vi "ExQSnapNframeSeq.vi"() -> ()   [LabVIEW 2010]
uses:
  Open-Close/CamHandle.vi
panel:
  out "Collecting":bool
  out "ADC Gain":u32
  out "ADC Offset":u32
  out "Pixel time":u32
  in  "OK Button":bool
  out "Readout Port":u32
  in  "ADC Gain":u32
  out "ADC Speed (Khz)":u32
  in  "ReadOut Port":u32 max=1 step=1
  in  "Trigger Edge":u32(ring)=1 items=["", "Positive (leading) edge", "Negative (falling) Edge"]
  in  "Trigger/Timing Mode":u32(ring)=1 items=["N/A", "FreeRun/Timed", "Single Trigger (PM only)", "Ext Sync/Strobed", "Bulb (PM only)", "Variable (PM only)", "Flash Mode (PM only)"]
  in  "Y End":u32=128 min=1 step=1
  in  "Y Start":u32=1 min=1 step=1
  in  "X Bin":u32=1 min=1 step=1
  in  "X End":u32=128 min=1 step=1
  in  "Y Bin":u32=1 min=1 step=1
  in  "X Start":u32=1 min=1 step=1
  in  "Number of Images":u32=50 min=1 step=1
  in  "Temperature":dbl format="%.2f"
  in  "Exposure":dbl min=0.0 step=0.001 format="%.3f"
  out "error out":errorcluster
  in  "error in (no error)":errorcluster
  # "ExCoolSnapNframeSeq:\nThis example sets up the camera with a given ROI, and \ncollects into a file \"number of Images\"  set by user. The \nImages are also displayed.\nNote: not all cameras support nframe.\nThis also shows how to setup the Cascade for nframe \nUsing Sequence mode"
  # "NOTICE\n\nTHIS VI USES A GLOBAL CAMERA HANDLE\n\nTHE VI EXOPENGLOBALCAM.VI MUST BE\nRUN AT THE START OF THE WORK SESSION.\nTHE CAMERA WILL REMAIN OPENED.\n\nTHE VI EXCLOSEGLOBALCAM.VI MUST\nBE RUN BEFORE LEAVING LABVIEW."
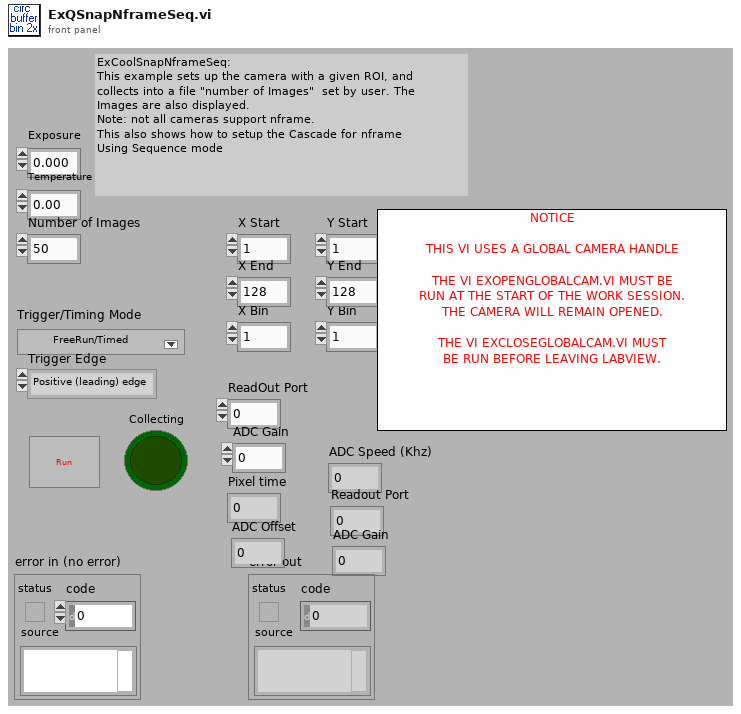
[diagram p1: front panel]
types:
  T1 = cluster{"X Start":u32, "X End":u32, "X Bin":u32, "Y Start":u32, "Y End":u32, "Y Bin":u32}
  T2 = cluster{"acquire focus mode":u32, "Exposure":dbl, "Number of Images":u32, "Software accumulation":u32}
  T3 = cluster{"Camera Handle":u32, "File Handle":u32, "Display Handle":u32, "Image Handle":u32}
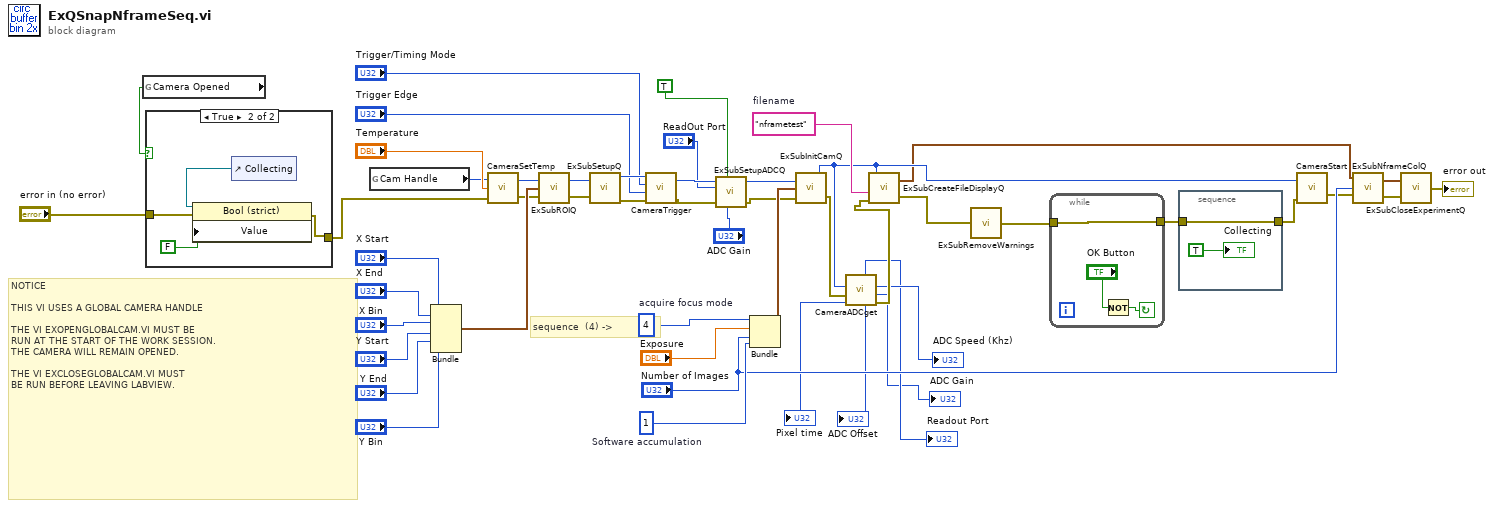
[diagram p0: block diagram]
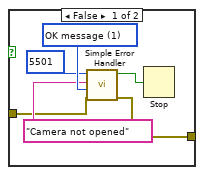
[diagram p2: hidden frame]
diagram:
  w44 = u32 4  # acquire focus mode
  w43 = u32 1  # Software accumulation
  w50 = "nframetest"  # filename
  # "NOTICE\n\nTHIS VI USES A GLOBAL CAMERA HANDLE\n\nTHE VI EXOPENGLOBALCAM.VI MUST BE\nRUN AT THE START OF THE WORK SESSION.\nTHE CAMERA WILL REMAIN OPENED.\n\nTHE VI EXCLOSEGLOBALCAM.VI MUST\nBE RUN BEFORE LEAVING LABVIEW."
  # "sequence  (4) ->"
  n1 = global read "CamHandle.vi" "Camera Opened"() -> (w7:bool)
  n2 = case shown="True" w7 {
    tunnel: [w55 w59] -> w5
    tunnel: "error in (no error)" -> [w51 w60]
    frame False {
      w56 = u16 1 items=["no dialog", "OK message", "continue or stop message"] ("type of dialog (OK msg:1)")
      n3 = call <vilib>:"Simple Error Handler.vi"("error code (no error:0)"=5501, "error source (\" \")"="Camera not opened", "type of dialog (OK msg:1)"=w56, "error in (no error)"=w51) -> ("error?"=w53:bool, "error out"=w55:errorcluster)  [unwired: 1 in, 3 out]
      n4 = Stop(stop? (T)=w53) -> ()
    }
    frame True {
      n5 = control-ref of="Collecting"() -> (w58:refnum<vi>)
      n6 = property class="Bool (strict)"(reference=w58, error in=w60, "Value"=FALSE) -> (error out=w59:errorcluster)  [unwired: 1 out]
    }
  }
  n7 = global read "CamHandle.vi" "Cam Handle"() -> (w4:u32)
  n8 = Bundle("X Start"="X Start", "X End"="X End", "X Bin"="X Bin", "Y Start"="Y Start", "Y End"="Y End", "Y Bin"="Y Bin") -> (w33:T1)  [unwired: 1 in]
  n9 = call <userlib>:"CameraSetTemp.vi"("error in (no error)"=w5, "Temperature"="Temperature", "Camera Handle"=w4) -> ("error out"=w30:errorcluster, "Camera Handle"=w31:u32)
  n10 = call "ExSubROIQ.vi"("error in (no error)"=w30, "ROI"=w33, "Camera Handle"=w31) -> ("error out"=w27:errorcluster, "Camera Handle"=w28:u32)
  n11 = call "ExSubSetupQ.vi"("error in (no error)"=w27, "Camera Handle"=w28) -> ("error out"=w45:errorcluster, "Camera Handle"=w46:u32)
  n12 = call <userlib>:"CameraTrigger.vi"("error in"=w45, "Trigger Edge"="Trigger Edge", "Timing Mode"="Trigger/Timing Mode", "Camera Handle"=w46) -> ("error out"=w23:errorcluster, "Camera Handle"=w24:u32)
  n13 = call "ExSubSetupADCQ.vi"("Camera Handle"=w24, "Fast ADC"=TRUE, "ReadOut Port"="ReadOut Port", "error in (no error)"=w23, "ADC Gain"="ADC Gain") -> ("Camera Handle"=w20:u32, "error out"=w19:errorcluster)  [unwired: 1 out]
  n14 = Bundle("acquire focus mode"=w44, "Exposure"="Exposure", "Number of Images"="Number of Images", "Software accumulation"=w43) -> (w48:T2)  [unwired: 1 in]
  n15 = call "ExSubInitCamQ.vi"("error in (no error)"=w19, "Camera Information"=w48, "Camera Handle"=w20) -> ("error out"=w17:errorcluster, "Camera Handle"=w14:u32)
  n16 = call <userlib>:"CameraADCget.vi"("Camera handle"=w14, "error in (no error)"=w17) -> ("Pixel Time"=→"Pixel time":i32, "Readout Port"=→"Readout Port":i32, "ADC Offset"=→"ADC Offset":i32, "ADC Speed"=→"ADC Speed (Khz)":i32, "ADC Gain"=→"ADC Gain":i32, "error out"=w16:errorcluster)  [unwired: 2 out]
  n17 = call "ExSubCreateFileDisplayQ.vi"("error in (no error)"=w16, "File and Display Name"=w50, "Camera Handle"=w14) -> ("error out"=w9:errorcluster, "Handles Out"=w1:T3)  [unwired: 1 in]
  n18 = call "ExSubRemoveWarnings.vi"("error in (no error)"=w9) -> ("error out"=w8:errorcluster)
  n19 = while {
    tunnel: [w63] -> w3
    tunnel: w8 -> [w63]
    stop <- w62 continue-if-true
    n20 = Not(x="OK Button") -> (.not. x?=w62:bool)
  }
  n21 = stacked-sequence {
    tunnel: w3 -> [w65]
    tunnel: [w65] -> w2
    frame #0 {
      "Collecting" <- TRUE
    }
  }
  n22 = call <userlib>:"CameraStart.vi"("error in"=w2, "Camera Handle"=w14) -> ("error out"=w32:errorcluster)  [unwired: 1 out]
  n23 = call "ExSubNframeColQ.vi"("error in (no error)"=w32, "Number of Images"="Number of Images", "Handle Cluster"=w1) -> ("error out"=w41:errorcluster, "Handle Cluster"=w42:T3)
  n24 = call "ExSubCloseExperimentQ.vi"("error in (no error)"=w41, "Handles In"=w42) -> ("error out"=→"error out":errorcluster)
